vi "Remove FP Menus.vi"(8 "error in (no error)":errorcluster, 11 "Main Window in":refnum<class "Main Window.lvclass">) -> (0 "error out":errorcluster, 3 "Main Window out":refnum<class "Main Window.lvclass">)   [LabVIEW 2021, in "Recipe.lvlib" / "Main Window.lvclass"]
uses:
  Main Window.lvclass
  Main Window.lvclass/Main Window.ctl
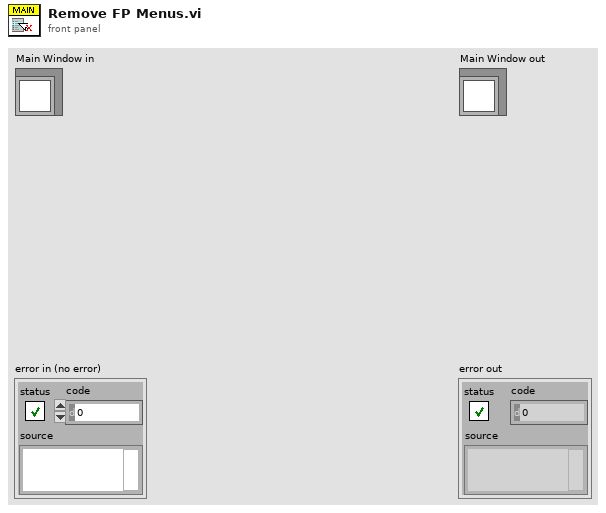
[diagram p1: front panel]
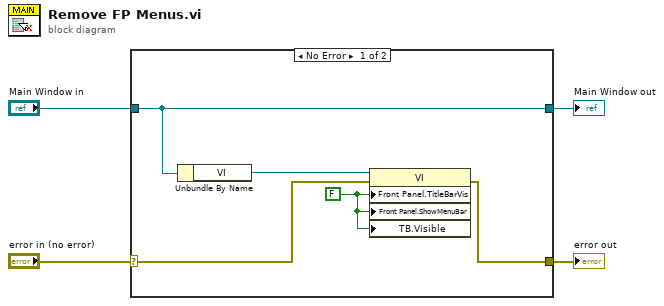
[diagram p0: block diagram]
diagram:
  n1 = case shown="No Error" "error in (no error)" {
    selector: "error in (no error)" -> [w8 w11]
    tunnel: [w7 w11] -> w3
    tunnel: [w6 w10] -> w1
    tunnel: "Main Window in" -> [w6 w10]
    frame No Error {
      w9 = FALSE ("Front Panel Window:Title Bar Visible")
      n2 = Unbundle By Name(w6) -> ("VI"=w5:refnum<vi>)
      n3 = property class="VI"(reference=w5, error in=w8, "Front Panel.TitleBarVis"=w9, "Front Panel.ShowMenuBar"=w9, "TB.Visible"=w9) -> (error out=w7:errorcluster)  [unwired: 1 out]
    }
    frame Error {
    }
  }
  "error out" <- w3
  "Main Window out" <- w1
